vi "reset_data.vi"(8 "error in (no error)":errorcluster, 11 "Experiment in":refnum<class "Experiment.lvclass">) -> (0 "error out":errorcluster, 3 "Experiment out":refnum<class "Experiment.lvclass">)   [LabVIEW 2013, in "Experiment.lvclass"]
uses:
  Experiment.lvclass
  Experiment.lvclass/Experiment.ctl
  TTL_input/TTL_input.lvclass
  Globals.vi
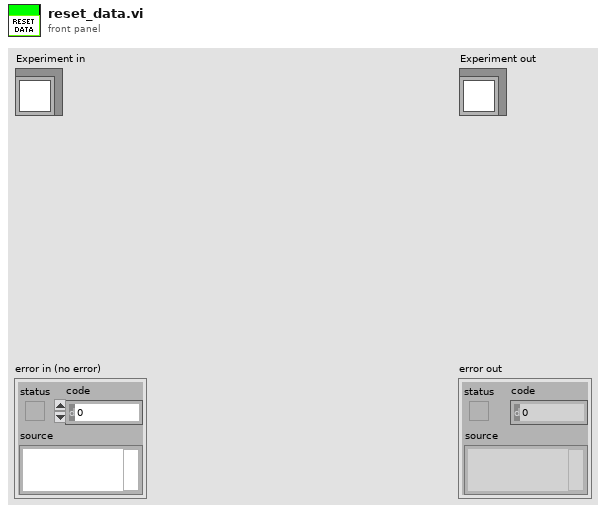
[diagram p1: front panel]
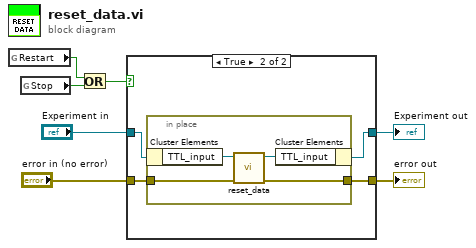
[diagram p0: block diagram]
diagram:
  n1 = global read "Globals.vi" "Restart"() -> (w2:bool)
  n2 = global read "Globals.vi" "Stop"() -> (w3:bool)
  n3 = Or(x=w2, y=w3) -> (x .or. y?=w1:bool)
  n4 = case shown="True" w1 {
    tunnel: [w9 w12] -> w6
    tunnel: "Experiment in" -> [w9 w13]
    tunnel: "error in (no error)" -> [w8 w11]
    tunnel: [w8 w10] -> w4
    frame False {
    }
    frame True {
      n5 = in-place {
        in-place-border: w11 -> [w15]
        in-place-border: [w14] -> w10
        n6 = in-place-cluster #1(w13) -> ("TTL_input"=w17:refnum<class "TTL_input.lvclass">)
        n7 = call-dynamic "reset_data.vi"("error in (no error)"=w15, "TTL_input in"=w17) -> ("error out"=w14:errorcluster, "TTL_input out"=w16:refnum<class "TTL_input.lvclass">)  [unwired: 8 in]
        n8 = in-place-cluster #1("TTL_input"=w16) -> (w12:refnum<class "Experiment.lvclass">)
      }
    }
  }
  "error out" <- w4
  "Experiment out" <- w6
